vi "WriteDataQ.vi"(6 "IndPoint":i32, 8 "error in (no error)":errorcluster caption="entrée d'erreur (pas d'erreur)", 9 "DataIn":dbl[](array[numeric]), 10 "ScanParIn":dbl[](array[numeric]), 11 "Interface en entrée":refnum<class "Interface.lvclass"> caption="DNL_LabVIEW Object in") -> (0 "error out":errorcluster caption="sortie d'erreur", 1 "CrvIndex":i32, 2 "CurCrvPointInd":i32, 3 "Interface en sortie":refnum<class "Interface.lvclass"> caption="DNL_LabVIEW Object out")   [LabVIEW 2019, in "Interface.lvclass"]
uses:
  Interface.lvclass
  Interface.lvclass/Interface.ctl
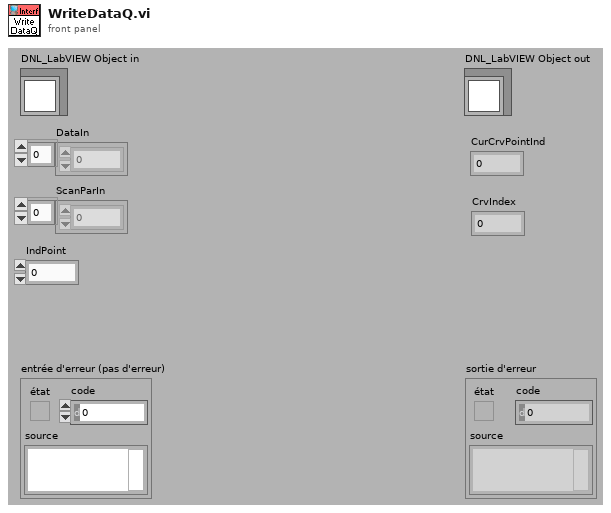
[diagram p1: front panel]
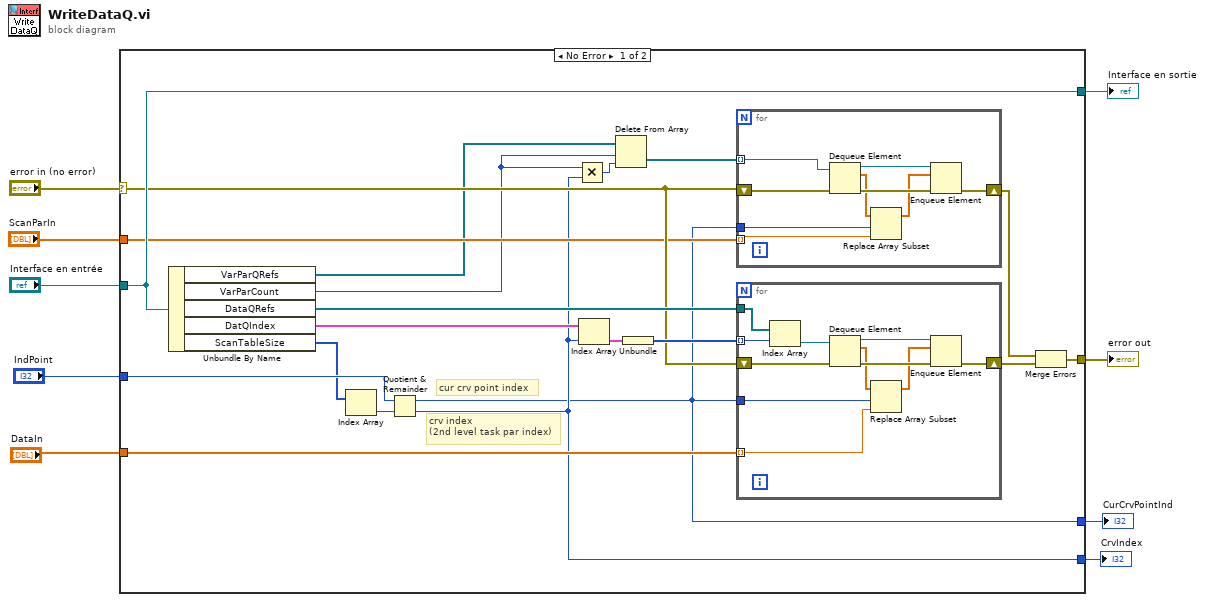
[diagram p0: block diagram]
diagram:
  n1 = case shown="No Error" "error in (no error)" {
    selector: "error in (no error)" -> [w19 w51]
    tunnel: [w18 w51] -> w8
    tunnel: [w27 w50] -> w6
    tunnel: "Interface en entrée" -> [w27 w50]
    tunnel: "DataIn" -> [w28 _]
    tunnel: "IndPoint" -> [w26 _]
    tunnel: [w10 _] -> w3
    tunnel: [w13 _] -> w2
    tunnel: "ScanParIn" -> [w16 _]
    frame No Error {
      # "crv index\n(2nd level task par index)"
      # "cur crv point index"
      n2 = Unbundle By Name(w27) -> ("VarParQRefs"=w15:refnum<queue>[], "VarParCount"=w12:i32, "DataQRefs"=w20:refnum<queue>[], "DatQIndex"=w24:cluster{"Tableau":i32[]}[], "ScanTableSize"=w25:i32[])
      n3 = Index Array(array=w25) -> (element=w22:i32)  [unwired: 1 in]
      n4 = Quotient & Remainder(x=w26, y=w22) -> (x-y*floor(x/y)=w10:i32, floor(x/y)=w13:i32)
      n5 = Multiply(x=w12, y=w13) -> (x*y=w14:i32)
      n6 = Index Array(array=w24, index=w13) -> (element=w21:cluster{"Tableau":i32[]})
      n7 = Delete From Array(array=w15, length=w12, index=w14) -> (deleted portion=w11:refnum<queue>[])  [unwired: 1 out]
      n8 = Unbundle(w21) -> ("Tableau"=w23:i32[])
      n9 = for {
        shift-right: [w37] -> w17
        shift-left: w19 -> [w31]
        tunnel: w16 -> [w33] mode=indexing
        tunnel: w10 -> [w32]
        tunnel: w11 -> [w30] mode=indexing
        n10 = Dequeue Element(queue=w30, error in (no error)=w31) -> (queue out=w38:refnum<queue>, element=w35:dbl[], error out=w36:errorcluster)  [unwired: 1 in, 1 out]
        n11 = Replace Array Subset(array=w35, new element=w33, index=w32) -> (w34:dbl[])
        n12 = Enqueue Element(queue=w38, element=w34, error in (no error)=w36) -> (error out=w37:errorcluster)  [unwired: 1 in, 2 out]
      }
      n13 = for {
        shift-right: [w48] -> w29
        shift-left: w19 -> [w42]
        tunnel: w28 -> [w44] mode=indexing
        tunnel: w10 -> [w43]
        tunnel: w20 -> [w41]
        tunnel: w23 -> [w40] mode=indexing
        n14 = Index Array(array=w41, index=w40) -> (element=w39:refnum<queue>)
        n15 = Dequeue Element(queue=w39, error in (no error)=w42) -> (queue out=w49:refnum<queue>, element=w46:dbl[], error out=w47:errorcluster)  [unwired: 1 in, 1 out]
        n16 = Replace Array Subset(array=w46, new element=w44, index=w43) -> (w45:dbl[])
        n17 = Enqueue Element(queue=w49, element=w45, error in (no error)=w47) -> (error out=w48:errorcluster)  [unwired: 1 in, 2 out]
      }
      n18 = Merge Errors(w17, w29) -> (w18:errorcluster)
    }
    frame Error {
    }
  }
  "error out" <- w8
  "Interface en sortie" <- w6
  "CurCrvPointInd" <- w3
  "CrvIndex" <- w2
